vi "Point in Polygon (Array).vi"(6 "tolerance":dbl=1e-09, 8 "Polygon Y":dbl[](array[numeric]), 9 "Polygon X":dbl[](array[numeric]), 10 "Y":dbl[](array[numeric]), 11 "X":dbl[](array[numeric])) -> (0 "error":i32, 3 "Position":T1[](array[typedef]) items=["Inside", "On Boundary", "Outside"])   [LabVIEW 2017, in "NI_AAL_Geometry.lvlib"]
doc: "Verifies whether a point is inside a polygon."
uses:
  <vilib>/Analysis/NI_AAL_Geometry.lvlib
  <vilib>/Analysis/geometry.llb/Point in Polygon Position.ctl
panel:
  # "Point in Polygon (Array)"
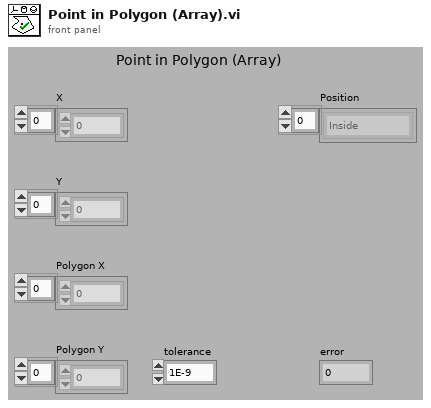
[diagram p1: front panel]
types:
  T1 = typedef "NI_AAL_Geometry.lvlib/Point in Polygon Position.ctl" = u16
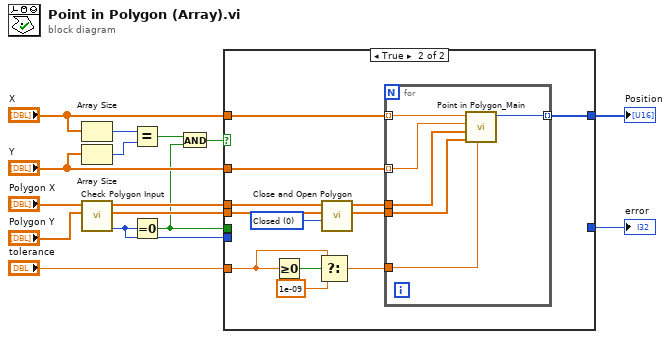
[diagram p0: block diagram]
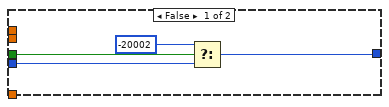
[diagram p2: hidden frame]
diagram:
  n1 = Array Size(array="X") -> (size(s)=w13:i32)
  n2 = Array Size(array="Y") -> (size(s)=w12:i32)
  n3 = call <vilib>:"Check Polygon Input.vi"("Y In"="Polygon Y", "X In"="Polygon X") -> ("error"=w1:i32, "Y Out"=w5:dbl[], "X Out"=w6:dbl[])  [unwired: 7 in]
  n4 = Equal?(x=w13, y=w12) -> (x = y?=w4:bool)
  n5 = Equal To 0?(x=w1) -> (x = 0?=w2:bool)
  n6 = And(x=w4, y=w2) -> (x .and. y?=w3:bool)
  n7 = case shown="True" w3 {
    tunnel: "X" -> [_ w31]
    tunnel: "Y" -> [_ w30]
    tunnel: w6 -> [_ w23]
    tunnel: w5 -> [_ w22]
    tunnel: [_ w29] -> w11
    tunnel: [w16 _] -> w10
    tunnel: "tolerance" -> [_ w26]
    tunnel: w2 -> [w19 _]
    tunnel: w1 -> [w17 _]
    frame False {
      n8 = Select(t=-20002, s=w19, f=w17) -> (s? t:f=w16:i32)
    }
    frame True {
      w24 = u16 0 items=["Closed", "Open"] ("type")
      n9 = Greater Or Equal To 0?(x=w26) -> (x >= 0?=w27:bool)
      n10 = Select(t=w26, s=w27, f=1e-09) -> (s? t:f=w25:dbl)
      n11 = call <vilib>:"Close and Open Polygon.vi"("type"=w24, "Y In"=w22, "X In"=w23) -> ("Y Out"=w20:dbl[], "X Out"=w21:dbl[])  [unwired: 7 in]
      n12 = for {
        tunnel: w31 -> [w37] mode=indexing
        tunnel: w30 -> [w36] mode=indexing
        tunnel: w21 -> [w35]
        tunnel: w20 -> [w34]
        tunnel: w25 -> [w33]
        tunnel: [w32] -> w29 mode=indexing
        n13 = call <vilib>:"Point in Polygon_Main.vi"("tolerance"=w33, "Polygon Y"=w34, "Polygon X"=w35, "y"=w36, "x"=w37) -> ("position"=w32:T1)  [unwired: 6 in]
      }
    }
  }
  "error" <- w10
  "Position" <- w11
